vi "unescape_special_characters.vi"(1 "String in":string) -> (0 "String out":string)   [LabVIEW 2015]
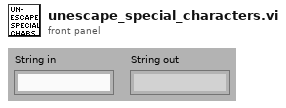
[diagram p1: front panel]
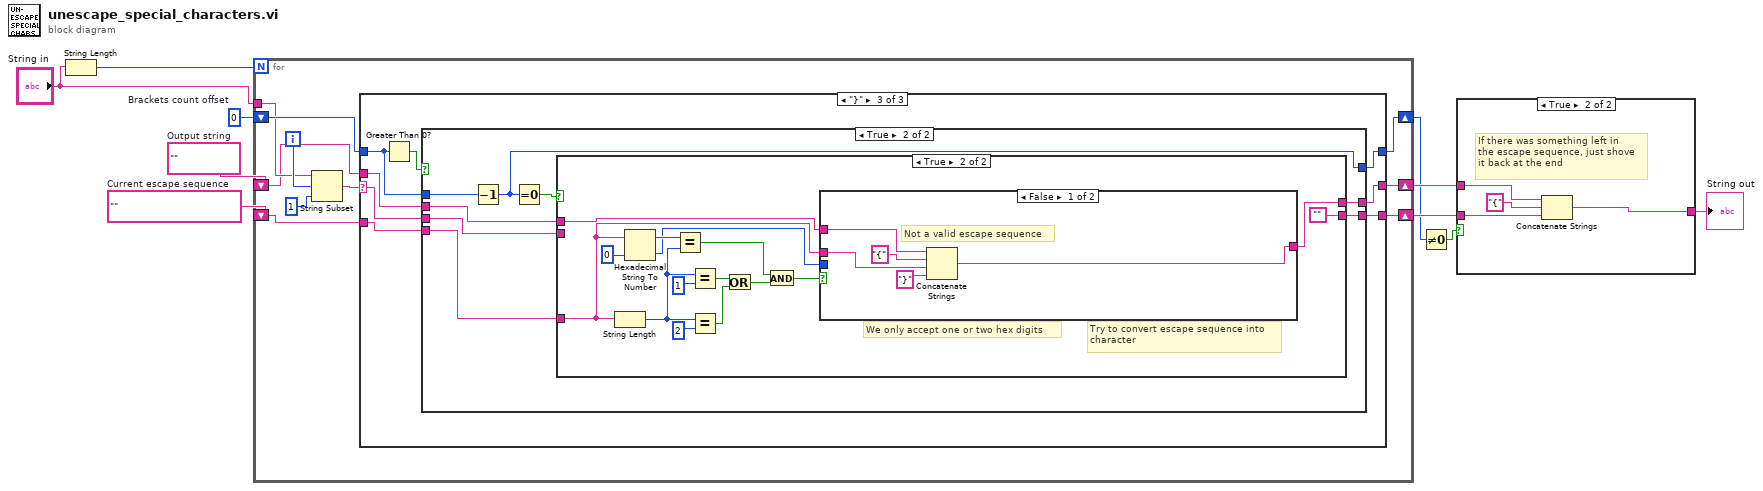
[diagram p0: block diagram]
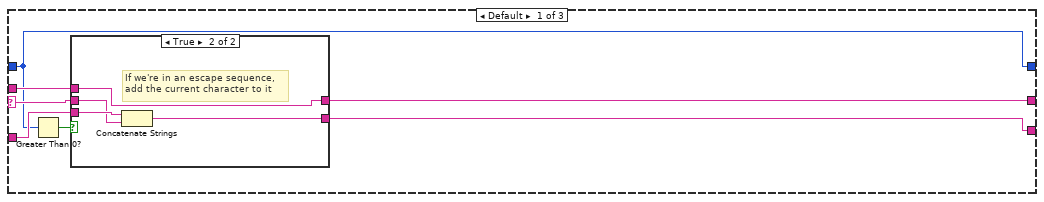
[diagram p3: hidden frame]
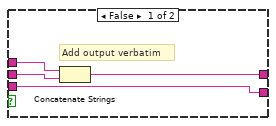
[diagram p4: hidden frame]
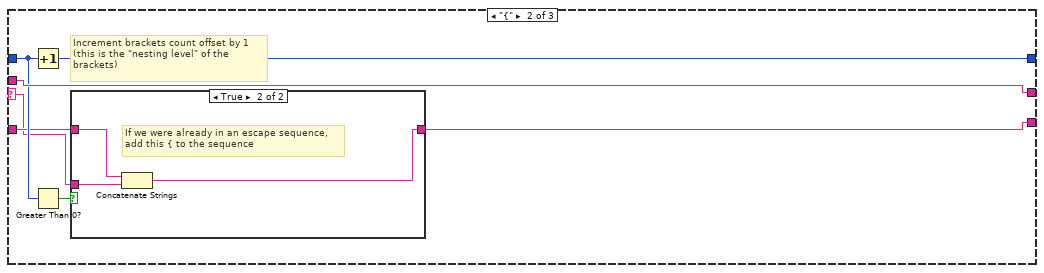
[diagram p5: hidden frame]
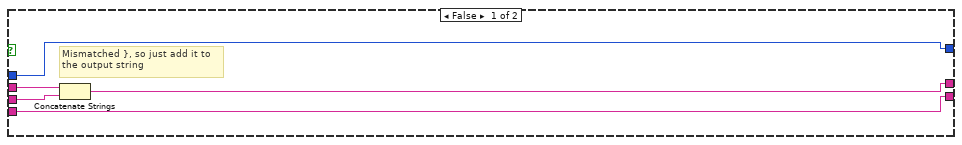
[diagram p7: hidden frame]
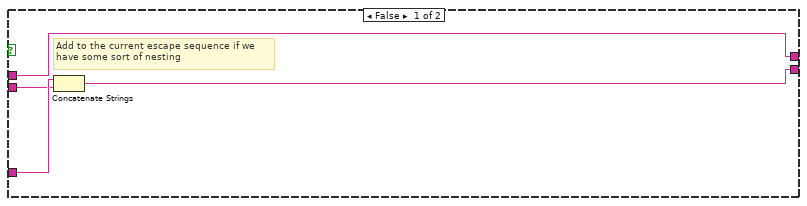
[diagram p8: hidden frame]
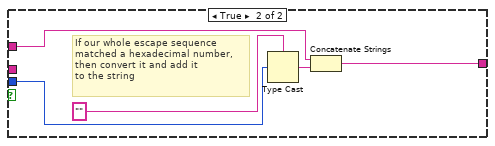
[diagram p9: hidden frame]
diagram:
  w7 = 0  # Brackets count offset
  w9 = ""  # Current escape sequence
  w10 = ""  # Output string
  n1 = String Length(string="String in") -> (length=w8:i32)
  n2 = for {
    N: w8 -> [_]
    shift-right: [w13] -> w5
    shift-left: w10 -> [w12]
    shift-right: [w15] -> w3
    shift-left: w9 -> [w16]
    shift-right: [w11] -> w1
    shift-left: w7 -> [w17]
    tunnel: "String in" -> [w14]
    i -> [w19]
    n3 = String Subset(string=w14, offset (0)=w19, length (rest)=1 ("length (rest)")) -> (substring=w18:string)
    n4 = case shown="\"}\"" w18 {
      selector: w18 -> [w25 w37 w47]
      tunnel: w17 -> [w21 w40 w53]
      tunnel: w16 -> [w26 w38 w51]
      tunnel: [w24 w36 w48] -> w15
      tunnel: w12 -> [w23 w41 w50]
      tunnel: [w22 w41 w49] -> w13
      tunnel: [w21 w42 w52] -> w11
      frame Default {
        n5 = Greater Than 0?(x=w21) -> (x > 0?=w27:bool)
        n6 = case shown="True" w27 {
          tunnel: w26 -> [w28 w35]
          tunnel: w25 -> [w30 w34]
          tunnel: [w28 w33] -> w24
          tunnel: w23 -> [w31 w32]
          tunnel: [w29 w32] -> w22
          frame False {
            # "Add output verbatim"
            n7 = Concatenate Strings(w31, w30) -> (w29:string)
          }
          frame True {
            # "If we're in an escape sequence,\nadd the current character to it"
            n8 = Concatenate Strings(w35, w34) -> (w33:string)
          }
        }
      }
      frame "{" {
        # "Increment brackets count offset by 1\n(this is the \"nesting level\" of the\nbrackets)"
        n9 = Increment(x=w40) -> (x+1=w42:i32)
        n10 = Greater Than 0?(x=w40) -> (x > 0?=w39:bool)
        n11 = case shown="True" w39 {
          tunnel: w38 -> [w43 w46]
          tunnel: w37 -> [_ w45]
          tunnel: [w43 w44] -> w36
          frame False {
          }
          frame True {
            # "If we were already in an escape sequence,\nadd this { to the sequence"
            n12 = Concatenate Strings(w46, w45) -> (w44:string)
          }
        }
      }
      frame "}" {
        n13 = Greater Than 0?(x=w53) -> (x > 0?=w54:bool)
        n14 = case shown="True" w54 {
          tunnel: w53 -> [w59 w67]
          tunnel: [w59 w66] -> w52
          tunnel: w51 -> [w55 w64]
          tunnel: w50 -> [w58 w63]
          tunnel: [w56 w62] -> w49
          tunnel: [w55 w61] -> w48
          tunnel: w47 -> [w57 w60]
          frame False {
            # "Mismatched }, so just add it to\nthe output string"
            n15 = Concatenate Strings(w58, w57) -> (w56:string)
          }
          frame True {
            n16 = Decrement(x=w67) -> (x-1=w66:i32)
            n17 = Equal To 0?(x=w66) -> (x = 0?=w65:bool)
            n18 = case shown="True" w65 {
              tunnel: w64 -> [w70 w77]
              tunnel: w63 -> [w71 w83]
              tunnel: [w71 w82] -> w62
              tunnel: [w68 ""] -> w61
              tunnel: w60 -> [w69 _]
              frame False {
                # "Add to the current escape sequence if we\nhave some sort of nesting"
                n19 = Concatenate Strings(w70, w69) -> (w68:string)
              }
              frame True {
                # "We only accept one or two hex digits"
                # "Try to convert escape sequence into\ncharacter"
                n20 = String Length(string=w77) -> (length=w72:i32)
                n21 = Hexadecimal String To Number(string=w77, default (0uL)=u8 0 ("default (0 U32)")) -> (offset past number=w85:i32, number=w84:u8)  [unwired: 1 in]
                n22 = Equal?(x=w85, y=w72) -> (x = y?=w80:bool)
                n23 = Equal?(x=w72, y=1) -> (x = y?=w76:bool)
                n24 = Equal?(x=w72, y=2) -> (x = y?=w73:bool)
                n25 = Or(x=w76, y=w73) -> (x .or. y?=w78:bool)
                n26 = And(x=w80, y=w78) -> (x .and. y?=w79:bool)
                n27 = case shown="False" w79 {
                  tunnel: w84 -> [_ w96]
                  tunnel: w83 -> [w91 w93]
                  tunnel: [w87 w92] -> w82
                  tunnel: w77 -> [w89 _]
                  frame False {
                    # "Not a valid escape sequence"
                    n28 = Concatenate Strings(w91, "{" ("string"), w89, "}" ("string")) -> (w87:string)
                  }
                  frame True {
                    # "If our whole escape sequence\nmatched a hexadecimal number,\nthen convert it and add it\nto the string"
                    n29 = Type Cast(type="", x=w96) -> (*(type *) &x=w94:string)
                    n30 = Concatenate Strings(w93, w94) -> (w92:string)
                  }
                }
              }
            }
          }
        }
      }
    }
  }
  n31 = Not Equal To 0?(x=w1) -> (x != 0?=w2:bool)
  n32 = case shown="True" w2 {
    tunnel: w5 -> [w97 w101]
    tunnel: [w97 w98] -> w4
    tunnel: w3 -> [_ w100]
    frame False {
    }
    frame True {
      # "If there was something left in\nthe escape sequence, just shove\nit back at the end"
      n33 = Concatenate Strings(w101, "{" ("string"), w100) -> (w98:string)
    }
  }
  "String out" <- w4
